vi "_036.vi"() -> ()   [LabVIEW 2024]
panel:
  out "Fibonacci series":i32[](array[numeric])
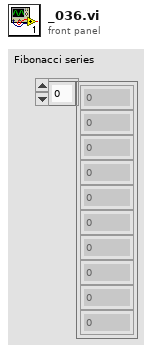
[diagram p1: front panel]
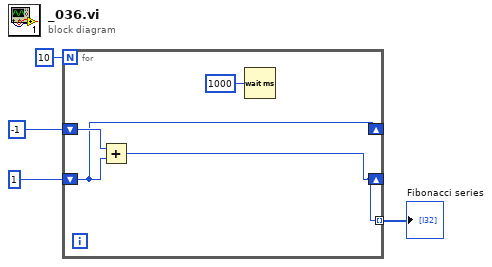
[diagram p0: block diagram]
diagram:
  n1 = for {
    N: 10 -> [_]
    shift-right: [w7] -> _
    shift-left: -1 -> [w8]
    shift-right: [w6] -> _
    shift-left: 1 -> [w7]
    tunnel: [w6] -> w1 mode=indexing
    n2 = Add(x=w8, y=w7) -> (x+y=w6:i32)
    n3 = Wait (ms)(milliseconds to wait=u32 1000) -> ()  [unwired: 1 out]
  }
  "Fibonacci series" <- w1
